vi "test Import Acyclic Frames.vi"(8 "error in":errorcluster, 11 "TestCase in":refnum<class "1553 Parameters Import.lvclass">) -> (0 "error out":errorcluster, 3 "TestCase out":refnum<class "1553 Parameters Import.lvclass">)   [LabVIEW 2020, in "1553 Parameters Import.lvclass"]
uses:
  1553 Parameters Import.lvclass
  Shared/Acyclic Frame Definition.ctl
  1553 Parameters Import.lvclass/1553 Parameters Import.ctl
  <vilib>/addons/_JKI Toolkits/VI Tester/TestCase.llb/TestCase.lvclass
  C:/Program Files (x86)/National Instruments/LabVIEW 2020/vi.lib/addons/_JKI Toolkits/VI Tester/TestCase.llb/TestCase.lvclass
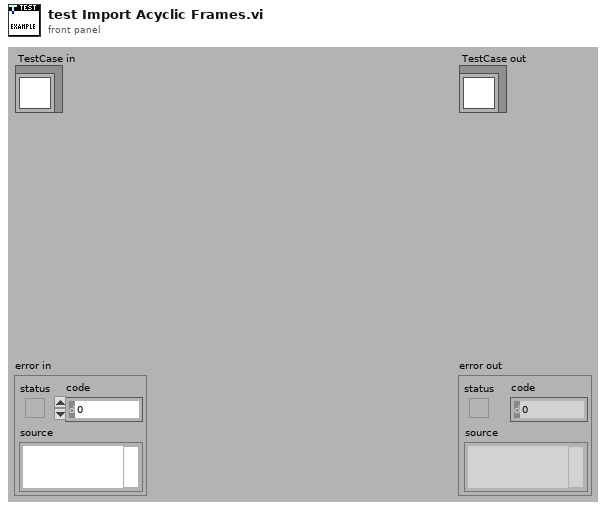
[diagram p1: front panel]
types:
  T1 = typedef "Acyclic Frame Definition.ctl" = cluster{"name":string, "messages":string[]}
  T2 = typedef "BIU Configuration.ctl" = cluster{"HW channel":u16, "terminal addresses":T3[], "terminal names":string[], "major frames":T4[], "minor frames":T5[], "acyclic frames":T1[], "messages":T6[]}
  T3 = typedef "Address.ctl" = u16
  T4 = typedef "Major Frame Definition.ctl" = cluster{"name":string, "minor frames":string[]}
  T5 = typedef "Minor Frame Definition.ctl" = cluster{"name":string, "messages":string[]}
  T6 = typedef "Message Definition.ctl" = cluster{"name":string, "message type":T7, "endpoint Tx":T8, "endpoint Rx":T8, "create timestamp channel":bool, "mode code":u16, "number of words":u16, "parameters":cluster{"name":string, "default value":dbl, "unit":string, "parameter definition":T9}[]}
  T7 = typedef "Message Type.ctl" = string
  T8 = typedef "Terminal Endpoint.ctl" = cluster{"terminal address":T3, "subaddress":T3}
  T9 = typedef "Parameter Definition.ctl" = cluster{"start index":i32, "size (bits)":i32, "encoding":enum16{"BNR", "BCD", "Discrete"}, "signed":bool, "multiplier":dbl, "offset":dbl}
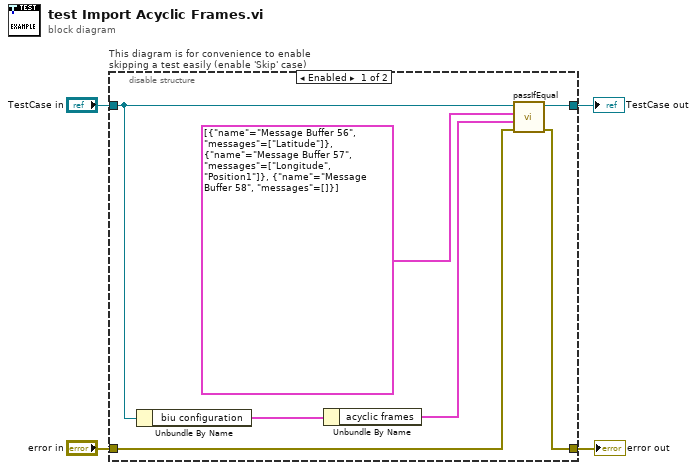
[diagram p0: block diagram]
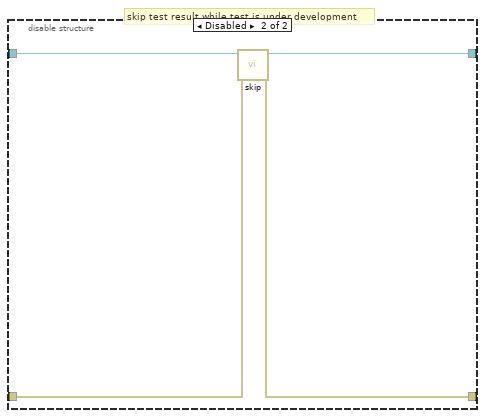
[diagram p2: hidden frame]
diagram:
  n1 = disable-structure "This diagram is for convenience to enable skipping a test easily (enable 'Skip' case)" shown="Enabled" {
    disable-tunnel: "TestCase in" -> [w9 w15]
    disable-tunnel: [w7 w13] -> w1
    disable-tunnel: [w6 w14] -> w3
    disable-tunnel: "error in" -> [w10 w12]
    frame Enabled {
      n2 = Unbundle By Name(w9) -> ("biu configuration"=w8:T2)
      n3 = Unbundle By Name(w8) -> ("acyclic frames"=w11:T1[])
      n4 = call-dynamic "passIfEqual.vi"("error in (no error)"=w10, "y"=w11, "x"=T1[] [{"name"="Message Buffer 56", "messages"=["Latitude"]}, {"name"="Message Buffer 57", "messages"=["Longitude", "Position1"]}, {"name"="Message Buffer 58", "messages"=[]}] ("acyclic frames"), "TestCase in"=w9) -> ("error out"=w6:errorcluster, "TestCase out"=w7:refnum<class "1553 Parameters Import.lvclass">)  [unwired: 6 in]
    }
    frame Disabled {
      # "skip test result while test is under development"
      n5 = call <vilib>:"skip.vi"("error in (no error)"=w12, "TestCase in"=w15) -> ("error out"=w14:errorcluster, "TestCase out"=w13:refnum<class "1553 Parameters Import.lvclass">)  [unwired: 8 in]
    }
  }
  "error out" <- w3
  "TestCase out" <- w1
